vi "Control System with Digital Twin.vi"() -> ()   [LabVIEW 2021]
uses:
  <vilib>/Simulation/Scripting/Companion Diagram/SimConfigNode/SimParams.ctl
  <vilib>/Simulation/Scripting/Companion Diagram/SimConfigNode/_simSolvers.ctl
  <vilib>/Simulation/Implementation/Shared/SIMSCR Execution Mode.ctl
  <vilib>/Simulation/Param Hierarchy/Typedefs/SIMPH Param Control Actions.ctl
  <vilib>/Simulation/Implementation/Shared/NILVSim_ParamChanged.vi
  <vilib>/Simulation/Implementation/Shared/NILVSIM_BeginStep.vi
  <vilib>/Simulation/Implementation/Shared/NILVSim_Manager.vi
  <vilib>/Utility/error.llb/Clear Errors.vi
  <vilib>/Simulation/Implementation/Shared/NILVSim_FinalizeModel.vi
  <vilib>/addons/control/pid/pid.llb/PID Advanced (DBL).vi
  <vilib>/Simulation/Implementation/Shared/SIM Unbundle Sim Info.vi
  <vilib>/Simulation/Implementation/Shared/NILVSim_Initialize.vi
  <vilib>/Simulation/Utility/Implementation/NILVSim Get Time and IsAcceptedStep.vi
  <vilib>/Simulation/Implementation/Shared/SIMSH Read Queue.vi
  <vilib>/Simulation/Implementation/Shared/NILVSim_GetModelError.vi
  <vilib>/Simulation/Implementation/Shared/SIM Bundle Sim Info.vi
  <vilib>/Simulation/Implementation/XNodeFramework/SimXNode/SimX.xnode
  Blackbox/Air Heater Black Box Model.vi
  <vilib>/Simulation/Scripting/Companion Diagram/SimConfigNode/SimDog.xnode
  SubVIs/Air Heater Model.vi
  <vilib>/addons/control/pid/NI_PID_pid.lvlib
  <vilib>/Simulation/Implementation/Shared/NI_SIM_Implementation.lvlib
panel:
  in  "LabVIEW PID SV [°C]":dbl=20.0 min=20.0 max=50.0 step=1.0
  out "Error [%]":dbl format="%.2g"
  out "Model [°C]":dbl format="%.2g"
  out "Control Chart":dbl(graph)=1.1724378087907898 caption="Controller Chart"
  in  "Model Parameters":T1={"T_init [C]"=21.1, "T [s]"=22.5, "K [C/V]"=3.9, "T_delay [s]"=2.1, "T_env [C]"=21.1}
  in  "LabVIEW PID Controller":cluster{"Kp":dbl, "Ti [s]":dbl, "Td [s]":dbl}={"Kp"=0.8, "Ti [s]"=20.0, "Td [s]"=0.0}
  in  "Stop Button":bool
  out "Measurement Chart":T2(graph)
  out "PV [°C]":dbl format="%.2g"
  out "MV [V]":dbl=1.0 format="%.2g"
  # "Process Value (PV)"
  # "Manipulated Value (MV)"
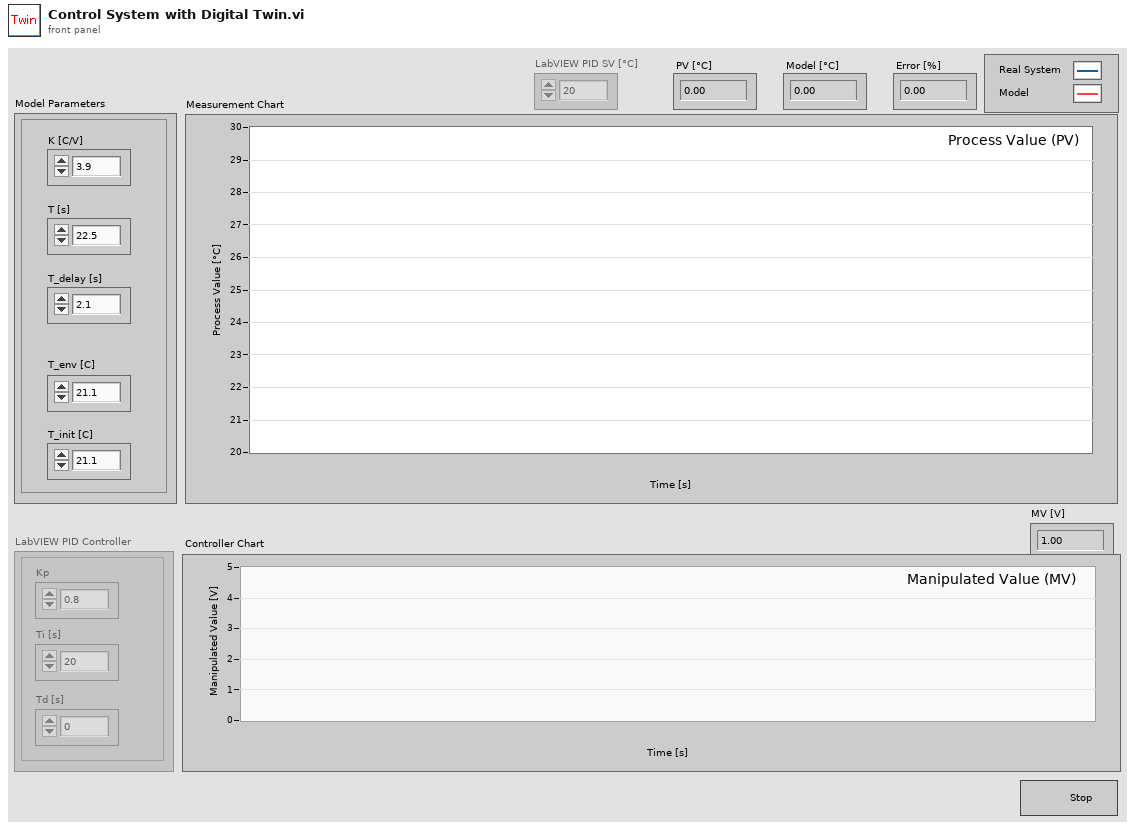
[diagram p1: front panel]
types:
  T1 = cluster{"T_init [C]":dbl, "T [s]":dbl, "K [C/V]":dbl, "T_delay [s]":dbl, "T_env [C]":dbl}
  T2 = cluster{"Output Value [20-50degC]":dbl, "Tout [C]":dbl}
  T3 = cluster{"Output Value [20-50degC]":dbl, "Tout [C]":dbl}[]
  T4 = enum16{"Simulate to Completion", "Single Time-Step Simulation (Fixed Step Only)"}
  T5 = typedef "SIMSCR Execution Mode.ctl" = enum16{"Simulate to Completion", "Single Time-Step Simulation (Fixed Step Only)"}
  T6 = typedef "SIMPH Param Control Actions.ctl" = enum16{"get params", "set params"}
  T7 = cluster{"SIMSH Sim Time":dbl, "Linear Scaling with Points.vi 2":cluster{"Output":dbl}, "Select":cluster{"s? t:f":dbl}, "Summation 3":cluster{"Result":dbl}, "Square Root":cluster{"sqrt(x)":dbl}, "Gaussian White Noise PtByPt.vi":cluster{"Gaussian white noise":dbl}, "Integrator":cluster{"output":dbl}, "Multiplication":cluster{"Result":dbl}, "Summation":cluster{"Result":dbl}, "Multiplication 2":cluster{"Result":dbl}, "Transport Delay":cluster{"output":dbl}, "Summation 2":cluster{"Result":dbl}}
  T8 = typedef "SimParams.ctl" = cluster{"Initial Time (s)":dbl, "Final Time (s)":dbl, "Step Size (s)":dbl, "ODE Solver":T9, "Minimum Step Size (s)":dbl, "Maximum Step Size (s)":dbl, "Relative Tolerance":dbl, "Absolute Tolerance":dbl, "Software Timing":bool, "Initial Step Size (s)":dbl, "Automatic Fixed Step Size?":bool, "Automatic Discrete Step Size?":bool, "Discrete Step Size (s)":dbl, "Calculate using Time Step":bool, "Solver Wired?":bool, "Prev.Frm.Expected End":u64, "Prev.Frm.Actual End":u64, "Prev.Frm.Finished Late?":bool, "Prev.Iter.Expected End":u64, "Prev.Iter.Actual End":u64, "Prev.Iter.Finished Late?":bool, "Expected Iteration Start":u64, "Actual Iteration Start":u64, "Expected Frame Start":u64, "Actual Frame Start":u64, "Source Name":string, "Name":string, "Period":i64, "Deadline":i64, "Offset":i64, "Start":i64, "Priority":i32, "Timeout":i32, "Processor":i32, "Mode":enum32{"No Change", "Process missed periods, maintain original phase", "Discard missed periods, maintain original phase", "Process missed periods, ignore original phase", "Discard missed periods, ignore original phase"}, "Wakeup reason":enum32{"Normal", "Aborted", "Asynchronous wakeup", "Timing source error", "Timed loop error", "Timeout"}, "Error":errorcluster, "Source Type":string, "Secondary Source Type":string, "Global End Time":u64, "Global Start Time":u64, "Full Solver Reset":bool, "Execution Mode":T5, "Nan/Inf Check":bool, "Custom Solver Library":string, "Solver Is Variable":bool, "custom solver name":string, "Signal Collection Decimation":u32}
  T9 = typedef "_simSolvers.ctl" = enum16{"Runge-Kutta 1 (Euler)", "Runge-Kutta 2", "Runge-Kutta 3", "Runge-Kutta 4", "Runge-Kutta 23 (variable)", "Runge-Kutta 45 (variable)", "BDF (variable)", "Adams-Moulton (variable)", "Rosenbrock (variable)", "Discrete States Only", "SDIRK 4 (variable)", "Radau 5 (variable)", "Radau 9 (variable)", "Radau 13 (variable)", "Radau [Variable Order] (variable)", "Gear's Method (variable)", "Linearizer", "State Query", "Trim Eval", "Custom Solver"}
  T10 = cluster{"SIMSH Sim Time":dbl, "lower limit":dbl, "Integrator":cluster{"output":dbl}, "Multiplication":cluster{"Result":dbl}, "Summation":cluster{"Result":dbl}, "Multiplication 2":cluster{"Result":dbl}, "Transport Delay":cluster{"output":dbl}, "Summation 2":cluster{"Result":dbl}}
  T11 = enum16{"LabVIEW PID", "Fuji PID Blackbox", "Real Fuji PID"}
  T12 = enum8{"Enabled", "Disabled", "Disabled and Grayed Out"}
  T13 = cluster{"Kp Scaling":dbl, "Ti Scaling":dbl, "Td Scaling":dbl}
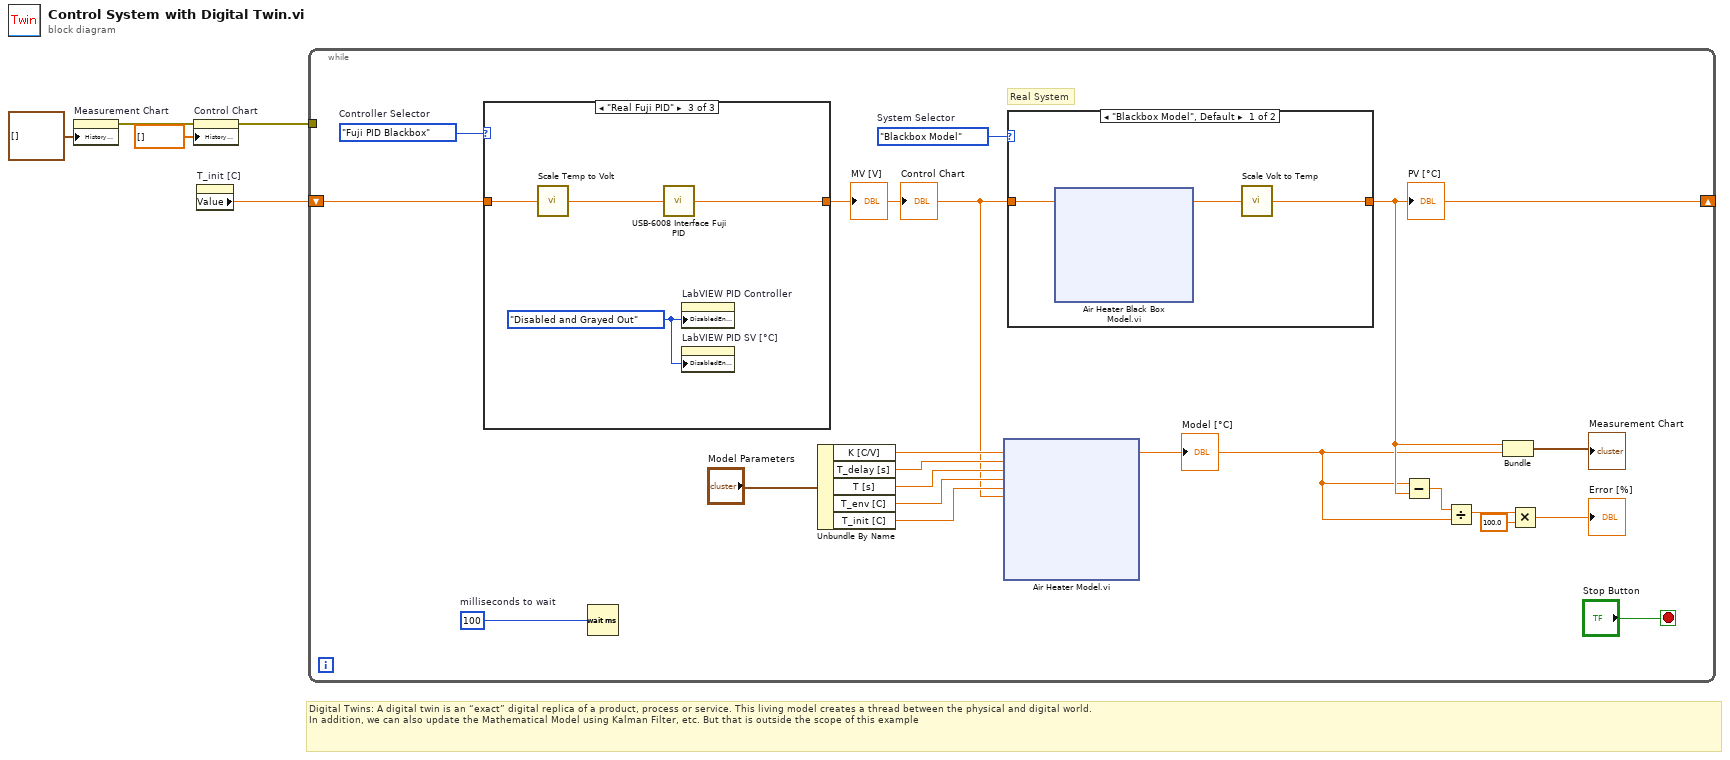
[diagram p0: block diagram]
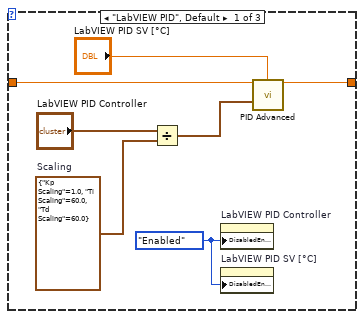
[diagram p2: hidden frame]
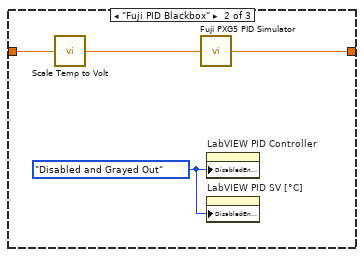
[diagram p3: hidden frame]
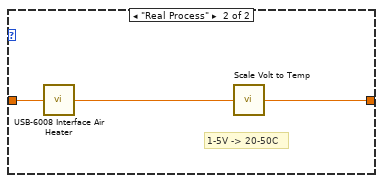
[diagram p4: hidden frame]
diagram:
  # "Digital Twins: A digital twin is an “exact” digital replica of a product, process or service. This living model creates a thread between the physical and digital world.\nIn addition, we can also update the Mathematical Model using Kalman Filter, etc. But that is outside the scope of this example"
  n1 = property on="Measurement Chart" class="WFChart (strict)"("History Data"=T3 []) -> (error out=w2:errorcluster)  [unwired: 2 in, 1 out]
  n2 = property on="Control Chart" class="WFChart (strict)"(error in=w2, "History Data"=dbl[] []) -> (error out=w1:errorcluster)  [unwired: 1 in, 1 out]
  n3 = property on="T_init [C]" class="DigNum (strict)"() -> ("Value"=w4:dbl)  [unwired: 2 in, 2 out]
  n4 = while {
    tunnel: w1 -> [_]
    shift-right: [w8] -> _
    shift-left: w4 -> [w22]
    stop <- "Stop Button" stop-if-true
    w6 = T11."Fuji PID Blackbox"  # Controller Selector
    w21 = enum16{"Blackbox Model", "Real Process"}."Blackbox Model"  # System Selector
    w23 = u32 100  # milliseconds to wait
    # "Real System"
    n5 = case shown="\"Real Fuji PID\"" w6 {
      tunnel: w22 -> [w31 w34 w39]
      tunnel: [w27 w35 w37] -> w13
      frame "LabVIEW PID", Default {
        w25 = T12."Enabled" ("Disabled")
        w29 = T13 {"Kp Scaling"=1.0, "Ti Scaling"=60.0, "Td Scaling"=60.0}  # Scaling
        n6 = Divide(x="LabVIEW PID Controller", y=w29) -> (x/y=w28:cluster{dbl, dbl, dbl})
        n7 = property on="LabVIEW PID Controller" class="Clust (strict)"("DisabledEnum"=w25) -> ()  [unwired: 2 in, 2 out]
        n8 = property on="LabVIEW PID SV [°C]" class="DigNum (strict)"("DisabledEnum"=w25) -> ()  [unwired: 2 in, 2 out]
        n9 = call-poly <vilib>:"PID Advanced.vi"("setpoint"="LabVIEW PID SV [°C]", "process variable"=w31, "PID gains"=w28) -> ("output"=w27:dbl)  [unwired: 11 in, 1 out]
      }
      frame "Fuji PID Blackbox" {
        w32 = T12."Disabled and Grayed Out" ("Disabled")
        n10 = call "Scale Temp to Volt.vi"("Input Value [20-50degC]"=w34) -> ("Output Value [1-5V]"=w33:dbl)
        n11 = call "Fuji PXG5 PID Simulator.vi"("Input (1-5V)"=w33) -> ("Output (0-5V)"=w35:dbl)
        n12 = property on="LabVIEW PID Controller" class="Clust (strict)"("DisabledEnum"=w32) -> ()  [unwired: 2 in, 2 out]
        n13 = property on="LabVIEW PID SV [°C]" class="DigNum (strict)"("DisabledEnum"=w32) -> ()  [unwired: 2 in, 2 out]
      }
      frame "Real Fuji PID" {
        w36 = T12."Disabled and Grayed Out" ("Disabled")
        n14 = call "Scale Temp to Volt.vi"("Input Value [20-50degC]"=w39) -> ("Output Value [1-5V]"=w38:dbl)
        n15 = call "USB-6008 Interface Fuji PID.vi"("Process Value  [1-5V]"=w38) -> ("Control Value [0-5V]"=w37:dbl)
        n16 = property on="LabVIEW PID Controller" class="Clust (strict)"("DisabledEnum"=w36) -> ()  [unwired: 2 in, 2 out]
        n17 = property on="LabVIEW PID SV [°C]" class="DigNum (strict)"("DisabledEnum"=w36) -> ()  [unwired: 2 in, 2 out]
      }
    }
    "MV [V]" <- w13
    "Control Chart" <- w13
    n18 = Wait (ms)(milliseconds to wait=w23) -> ()  [unwired: 1 out]
    n19 = Unbundle By Name("Model Parameters") -> ("K [C/V]"=w18:dbl, "T_delay [s]"=w17:dbl, "T [s]"=w16:dbl, "T_env [C]"=w15:dbl, "T_init [C]"=w14:dbl)
    n20 = xnode "Air Heater Model.vi"("K [C/V]"=w18, "T_delay [s]"=w17, "T [s]"=w16, "T_env [C]"=w15, "T_init [C]"=w14, "u [V]"=w13) -> ("Tout [C]"=w7:dbl)  [unwired: 2 in, 10 out]
    "Model [°C]" <- w7
    n21 = case shown="\"Blackbox Model\", Default" w21 {
      tunnel: w13 -> [w42 w290]
      tunnel: [w40 w288] -> w8
      frame "Blackbox Model", Default {
        n22 = xnode "Air Heater Black Box Model.vi"("Control Signal [0-5V]"=w42) -> ("Tout [1-5V]"=w41:dbl)  [unwired: 2 in, 1 out]
        n23 = call "Scale Volt to Temp.vi"("Input Value [1-5V]"=w41) -> ("Output Value [20-50degC]"=w40:dbl)
      }
      frame "Real Process" {
        # "1-5V -> 20-50C"
        n24 = call "USB-6008 Interface Air Heater.vi"("Control Signal [0-5V]"=w290) -> ("Process Value [1-5V]"=w289:dbl)
        n25 = call "Scale Volt to Temp.vi"("Input Value [1-5V]"=w289) -> ("Output Value [20-50degC]"=w288:dbl)
      }
    }
    "PV [°C]" <- w8
    n26 = Subtract(x=w7, y=w8) -> (x-y=w12:dbl)
    n27 = Divide(x=w12, y=w7) -> (x/y=w11:dbl)
    n28 = Bundle "Bundle"("Output Value [20-50degC]"=w8, "Tout [C]"=w7) -> (→"Measurement Chart":T2)  [unwired: 1 in]
    n29 = Multiply(x=w11, y=100.0) -> (x*y=→"Error [%]":dbl)
  }
